vi "pump.vi"() -> ()   [LabVIEW 2015]
uses:
  <vilib>/Plasmionique/MB Master/MB_Master_Serial/MB_Master_Serial.lvclass
  <vilib>/Plasmionique/MB Master/MB Master.lvlib
panel:
  out "Registers":u16[](array[numeric])
  in  "quantity":u16
  in  "Serial Config":T1={"baud rate (bps)"=19200, "stop bits"=10, "parity"=0, "flow control"=0, "timeout"=1000, "retries"=1} {"stop bits" items=["1.0"=10, "1.5"=15, "2.0"=20]; "flow control" items=["None", "XON/XOFF", "RTS/CTS", "XON/XOFF & RTS/CTS", "DTR/DSR", "XON/XOFF & DTR/DSR"]; "parity" items=["None", "Odd", "Even", "Mark", "Space"]}
  in  "address":u16
  out "error out":errorcluster
  in  "Error in":errorcluster caption="Error in (no error)"
  in  "Slave ID":u8=1
  in  "VISA resource name":refnum<visa-resource-name>
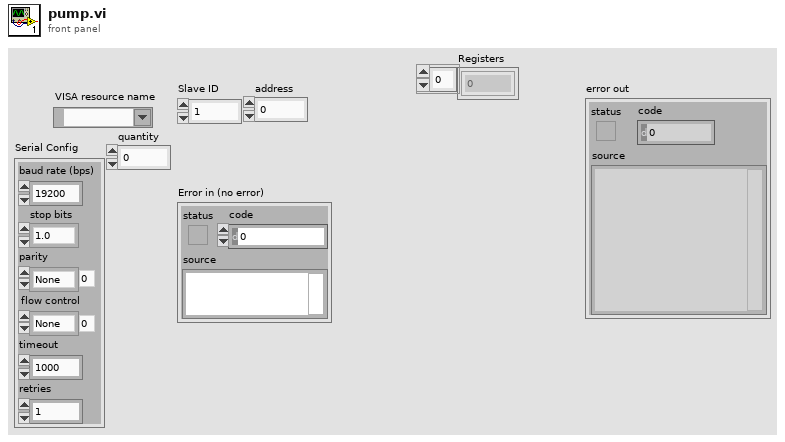
[diagram p1: front panel]
types:
  T1 = cluster{"baud rate (bps)":u32, "stop bits":u16, "parity":u16, "flow control":u16, "timeout":u32, "retries":i32}
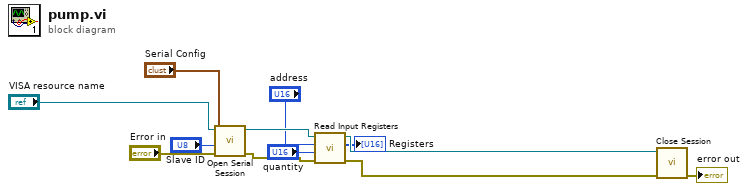
[diagram p0: block diagram]
diagram:
  n1 = call <vilib>:"Open Serial Session.vi"("Error in"="Error in", "Slave ID"="Slave ID", "Serial Config"="Serial Config", "VISA Resource"="VISA resource name") -> ("Error out"=w7:errorcluster, "MB_Serial session"=w4:refnum<class "MB_Master_Serial.lvclass">)  [unwired: 6 in]
  n2 = call <vilib>:"Read Input Registers.vi"("error in (no error)"=w7, "quantity"="quantity", "starting address"="address", "MB session in"=w4) -> ("error out"=w6:errorcluster, "Registers"=→"Registers":u16[], "MB session out"=w5:refnum<class "MB_Master_Serial.lvclass">)  [unwired: 5 in]
  n3 = call-dynamic "Close Session.vi"("error in (no error)"=w6, "MB_Serial session"=w5) -> ("error out"=→"error out":errorcluster)  [unwired: 9 in]
